vi "Read val.vi"(8 "error in (no error)":errorcluster, 11 "Switch DBL in":refnum<class "Switch DBL.lvclass">) -> (0 "error out":errorcluster, 2 "val":dbl, 3 "Switch DBL out":refnum<class "Switch DBL.lvclass">)   [LabVIEW 2016, in "Sequence Composition.lvlib" / "Switch DBL.lvclass"]
uses:
  Switch DBL.lvclass
  Switch DBL.lvclass/Switch DBL.ctl
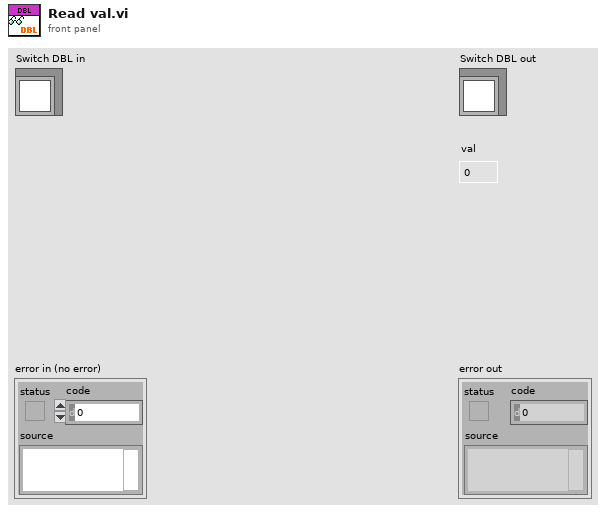
[diagram p1: front panel]
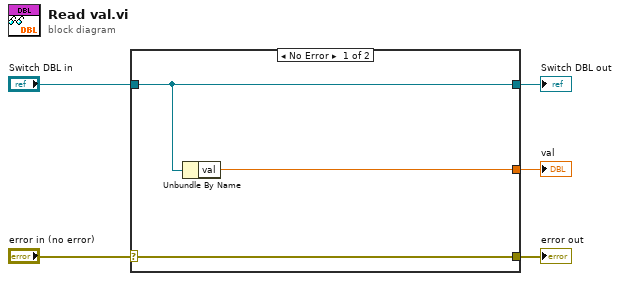
[diagram p0: block diagram]
diagram:
  n1 = case shown="No Error" "error in (no error)" {
    selector: "error in (no error)" -> [w8 w9]
    tunnel: [w8 w9] -> w4
    tunnel: [w7 w10] -> w2
    tunnel: "Switch DBL in" -> [w7 w10]
    tunnel: [w6 _] -> w1
    frame No Error {
      n2 = Unbundle By Name(w7) -> ("val"=w6:dbl)
    }
    frame Error {
    }
  }
  "error out" <- w4
  "Switch DBL out" <- w2
  "val" <- w1
